vi "pulse_generator_data_v2.vi"(3 "PG Data":refnum<vi>, 4 "Record dP Data":refnum<vi>, 5 "queue in":refnum<queue>, 6 "Stop! Refnum":refnum<vi>, 7 "Recording Progressbar":refnum<vi>, 8 "Seesion Start Time":timestamp, 9 "Pulse Generator Chart Refnums":T3, 10 "Pulse Generator Offsets and Data Saving Controls Refnums":T2, 11 "Pulse Generator Measurement Refnums":T1) -> ()   [LabVIEW 2017]
uses:
  pulse_generator_data_charts_refnums.ctl
  pulse_generator_data_controls_refnums.ctl
  pulse_generator_data_refnums.ctl
  <vilib>/Waveform/WDTOps.llb/WDT Get Waveform Time Array DBL.vi
panel:
  out "size(s)":i32[](graph)
  out "Sampling Rate":refnum<vi>
  out "Recording Duration":refnum<vi>
  out "Camera Voltage Chart":refnum<vi>
  out "Abs Tank Pressure Chart":refnum<vi>
  out "Pitot dP Chart":refnum<vi>
  out "Pulse Generator to Test Section dP Chart":refnum<vi>
  out "W1-7 dP":refnum<vi>
  out "W1-4 dP":refnum<vi>
  out "Mass Flow Rate":refnum<vi>
  out "Liquid Sat Pressure":refnum<vi>
  out "Liquid Temperature":refnum<vi>
  out "Vapor Sat Pressure":refnum<vi>
  out "Vapor Temperature":refnum<vi>
  out "Pitot dP":refnum<vi>
  out "PG to TS dP":refnum<vi>
  out "Pitot Current":refnum<vi>
  out "PG Abs Pressure":refnum<vi>
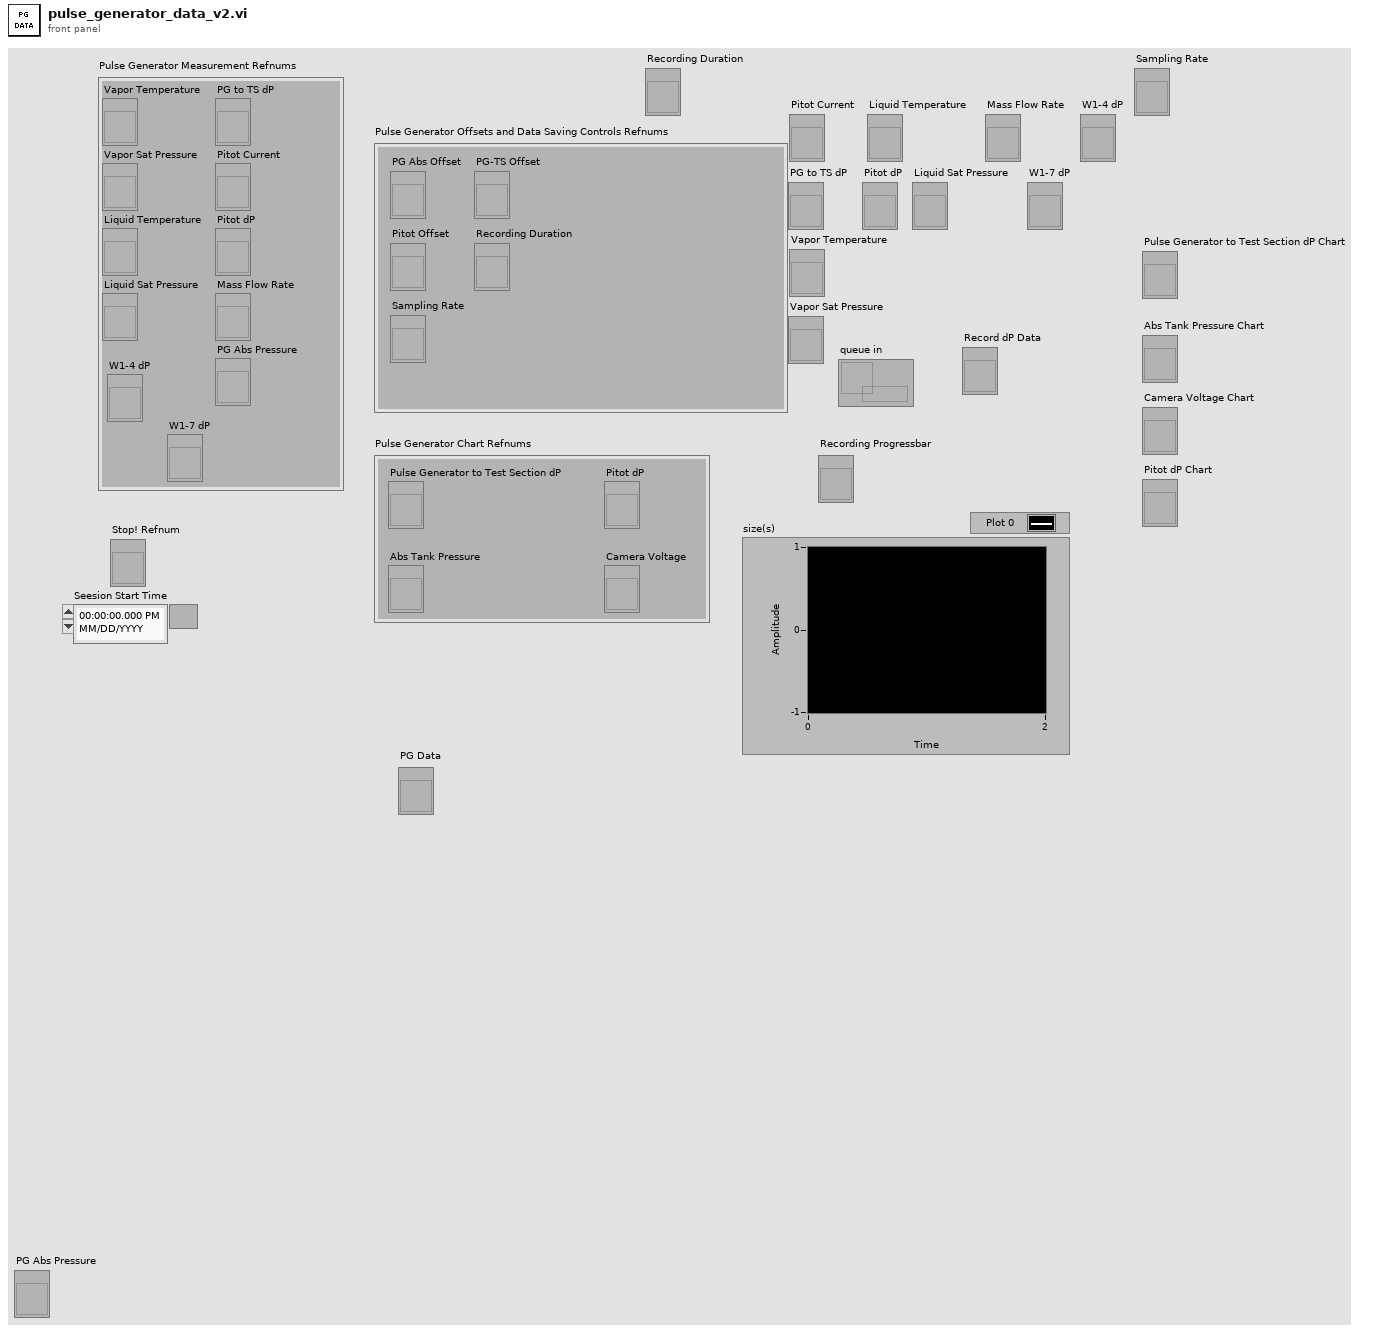
[diagram p1: front panel]
types:
  T1 = typedef "pulse_generator_data_refnums.ctl" = cluster{"Vapor Temperature":refnum<vi>, "Vapor Sat Pressure":refnum<vi>, "Liquid Temperature":refnum<vi>, "Liquid Sat Pressure":refnum<vi>, "PG to TS dP":refnum<vi>, "Pitot Current":refnum<vi>, "Pitot dP":refnum<vi>, "Mass Flow Rate":refnum<vi>, "PG Abs Pressure":refnum<vi>, "W1-4 dP":refnum<vi>, "W1-7 dP":refnum<vi>}
  T2 = typedef "pulse_generator_data_controls_refnums.ctl" = cluster{"PG Abs Offset":refnum<vi>, "Pitot Offset":refnum<vi>, "PG-TS Offset":refnum<vi>, "Recording Duration":refnum<vi>, "Sampling Rate":refnum<vi>}
  T3 = typedef "pulse_generator_data_charts_refnums.ctl" = cluster{"Pulse Generator to Test Section dP":refnum<vi>, "Pitot dP":refnum<vi>, "Abs Tank Pressure":refnum<vi>, "Camera Voltage":refnum<vi>}
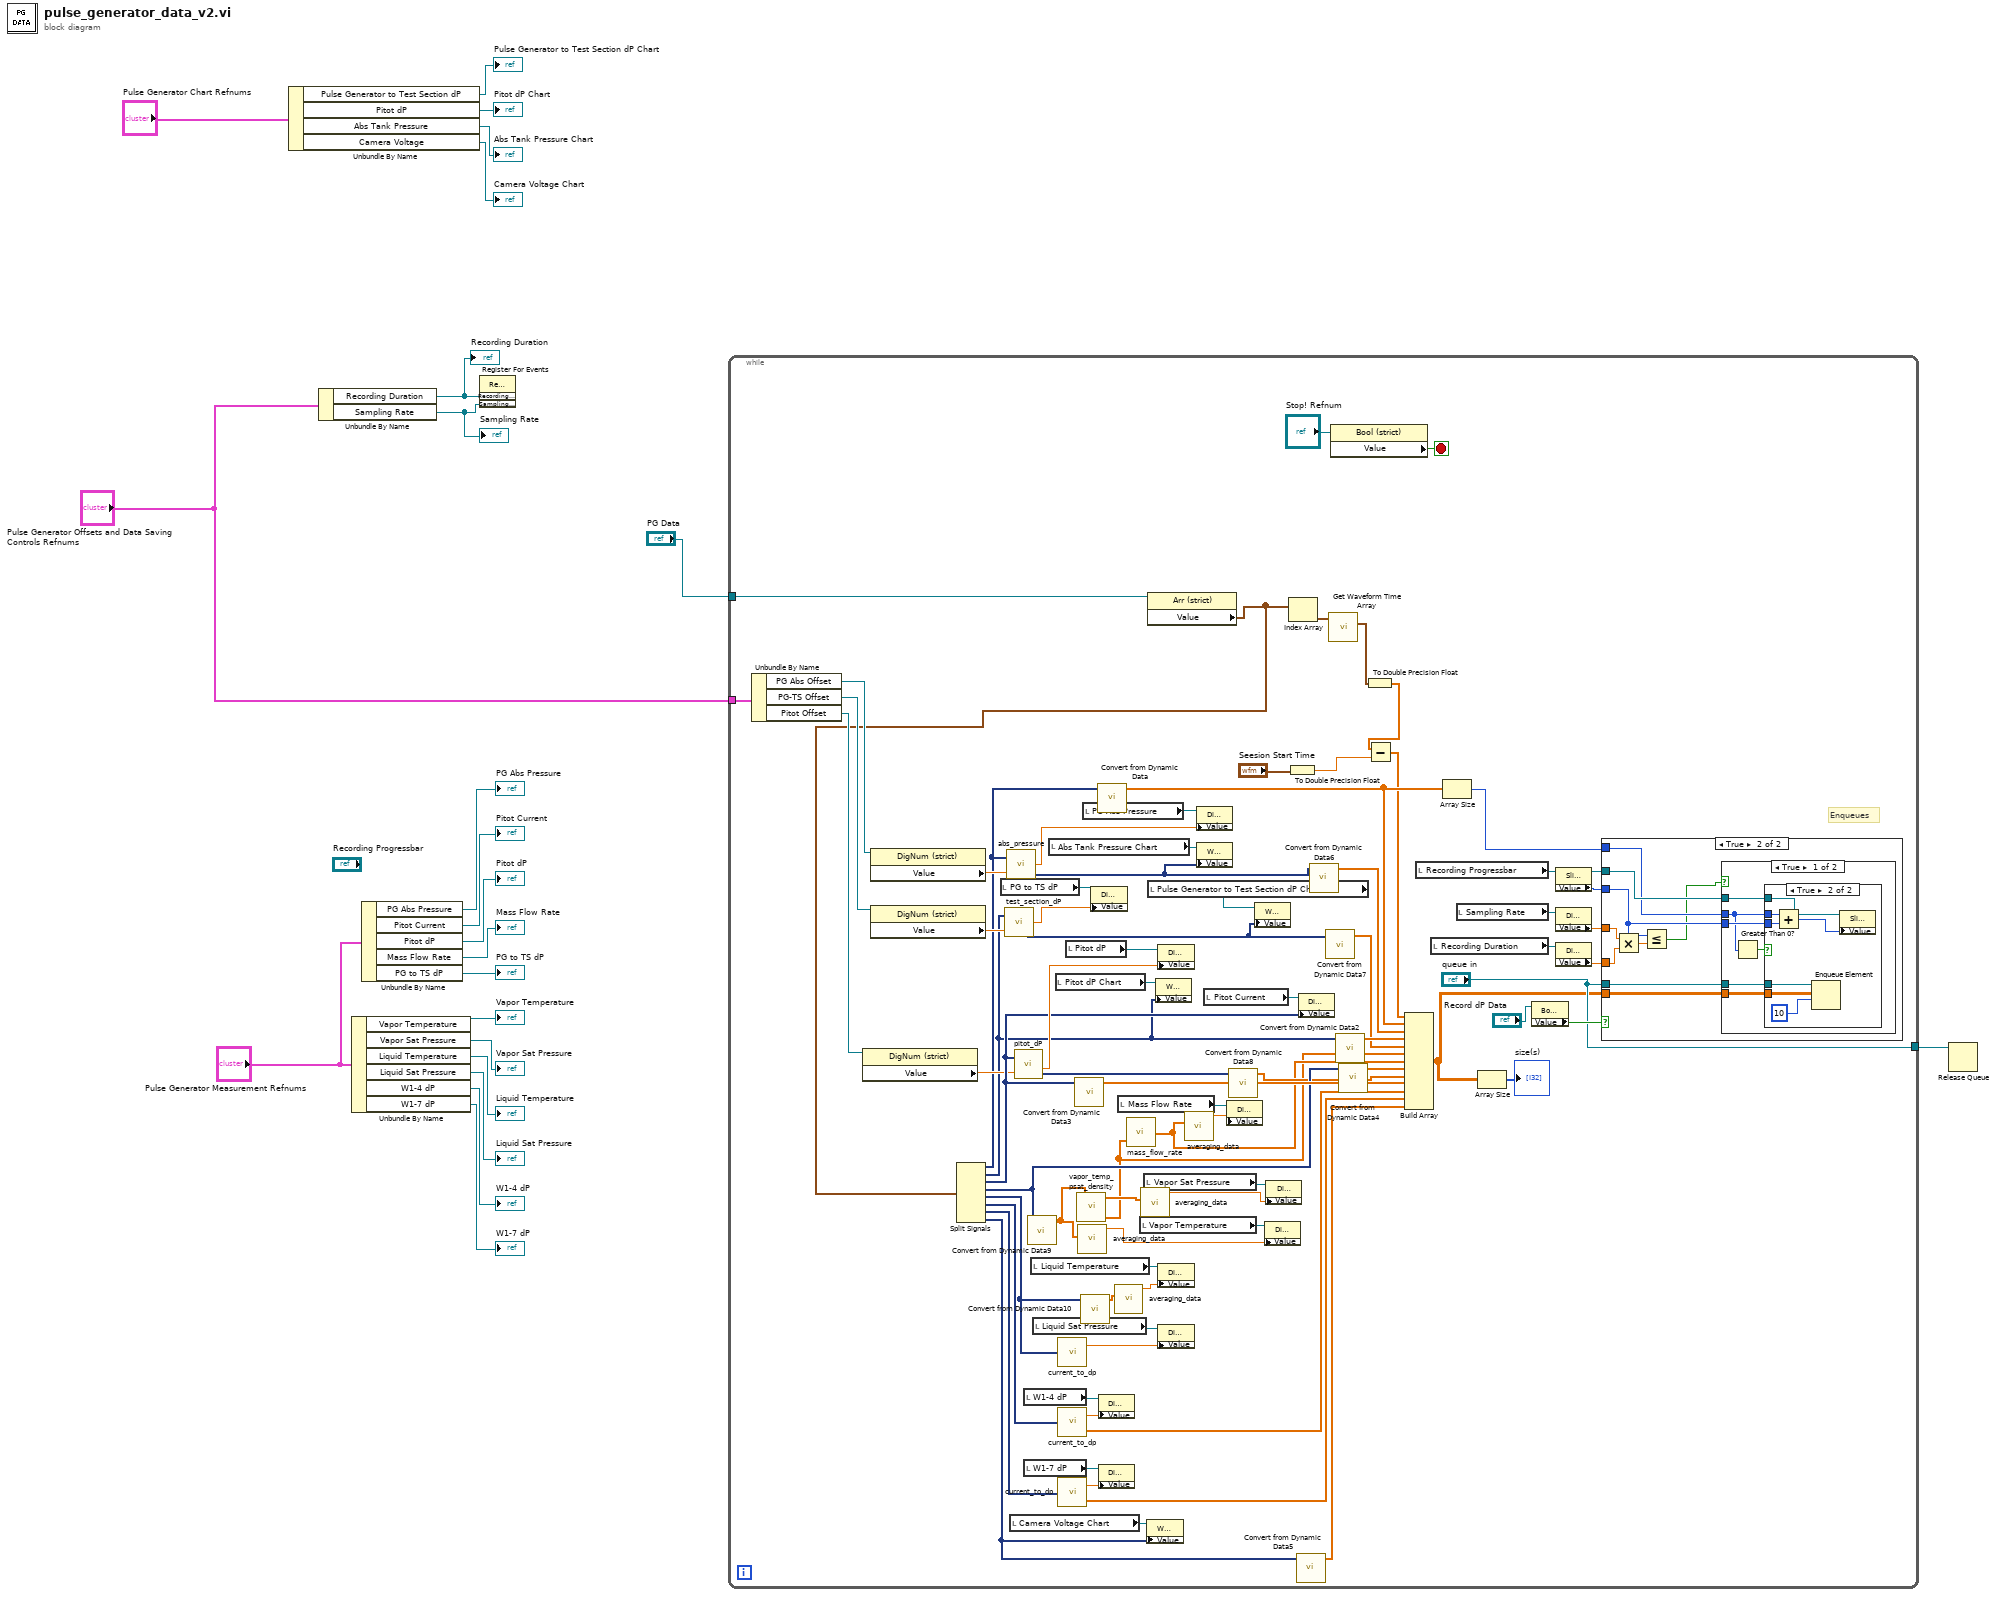
[diagram p0: block diagram]
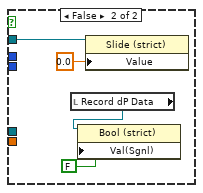
[diagram p4: hidden frame]
diagram:
  n1 = Unbundle By Name("Pulse Generator Chart Refnums") -> ("Pulse Generator to Test Section dP"=→"Pulse Generator to Test Section dP Chart":refnum<vi>, "Pitot dP"=→"Pitot dP Chart":refnum<vi>, "Abs Tank Pressure"=→"Abs Tank Pressure Chart":refnum<vi>, "Camera Voltage"=→"Camera Voltage Chart":refnum<vi>)
  n2 = Unbundle By Name("Pulse Generator Offsets and Data Saving Controls Refnums") -> ("Recording Duration"=w4:refnum<vi>, "Sampling Rate"=w3:refnum<vi>)
  "Recording Duration" <- w4
  "Sampling Rate" <- w3
  n3 = Unbundle By Name("Pulse Generator Measurement Refnums") -> ("Vapor Temperature"=→"Vapor Temperature":refnum<vi>, "Vapor Sat Pressure"=→"Vapor Sat Pressure":refnum<vi>, "Liquid Temperature"=→"Liquid Temperature":refnum<vi>, "Liquid Sat Pressure"=→"Liquid Sat Pressure":refnum<vi>, "W1-4 dP"=→"W1-4 dP":refnum<vi>, "W1-7 dP"=→"W1-7 dP":refnum<vi>)
  n4 = Unbundle By Name("Pulse Generator Measurement Refnums") -> ("PG Abs Pressure"=→"PG Abs Pressure":refnum<vi>, "Pitot Current"=→"Pitot Current":refnum<vi>, "Pitot dP"=→"Pitot dP":refnum<vi>, "Mass Flow Rate"=→"Mass Flow Rate":refnum<vi>, "PG to TS dP"=→"PG to TS dP":refnum<vi>)
  n5 = register-events(w4, w3) -> ()  [unwired: 2 in, 2 out]
  n6 = while {
    tunnel: "Pulse Generator Offsets and Data Saving Controls Refnums" -> [w101]
    tunnel: ["queue in"] -> w6
    tunnel: "PG Data" -> [w34]
    stop <- w102 stop-if-true
    # "Enqueues"
    n7 = Unbundle By Name(w101) -> ("PG Abs Offset"=w100:refnum<vi>, "PG-TS Offset"=w99:refnum<vi>, "Pitot Offset"=w98:refnum<vi>)
    n8 = property class="DigNum (strict)"(reference=w98) -> ("Value"=w52:dbl)  [unwired: 1 in, 2 out]
    n9 = property class="DigNum (strict)"(reference=w100) -> ("Value"=w97:dbl)  [unwired: 1 in, 2 out]
    n10 = property class="DigNum (strict)"(reference=w99) -> ("Value"=w56:dbl)  [unwired: 1 in, 2 out]
    n11 = local read "PG to TS dP"() -> (w96:refnum<vi>)
    n12 = local read "Camera Voltage Chart"() -> (w77:refnum<vi>)
    n13 = local read "W1-4 dP"() -> (w87:refnum<vi>)
    n14 = local read "W1-7 dP"() -> (w84:refnum<vi>)
    n15 = local read "Liquid Temperature"() -> (w90:refnum<vi>)
    n16 = local read "Liquid Sat Pressure"() -> (w92:refnum<vi>)
    n17 = local read "Abs Tank Pressure Chart"() -> (w80:refnum<vi>)
    n18 = local read "Pitot dP Chart"() -> (w79:refnum<vi>)
    n19 = local read "Pitot dP"() -> (w94:refnum<vi>)
    n20 = local read "PG Abs Pressure"() -> (w54:refnum<vi>)
    n21 = local read "Mass Flow Rate"() -> (w93:refnum<vi>)
    n22 = local read "Vapor Temperature"() -> (w89:refnum<vi>)
    n23 = local read "Vapor Sat Pressure"() -> (w82:refnum<vi>)
    n24 = property class="Arr (strict)"(reference=w34) -> ("Value"=w33:waveform(dbl)[])  [unwired: 1 in, 2 out]
    n25 = Split Signals(w33) -> (w41:dynamicdata, w50:dynamicdata, w59:dynamicdata, w57:dynamicdata, w28:dynamicdata, w86:dynamicdata, w85:dynamicdata, w68:dynamicdata)  [unwired: 8 in]
    n26 = call "test_section_dP.vi"("dP Voltage"=w50, "Offset[Pa]"=w56) -> ("Adj dP"=w75:dbl, "Adj dP Array"=w44:dynamicdata)  [unwired: 1 out]
    n27 = call "abs_pressure.vi"("Input Voltage"=w41, "Offset[Pa]"=w97) -> ("Adj Absolute Pressure"=w76:dbl, "Adj Absolute Pressure Array"=w46:dynamicdata)  [unwired: 1 out]
    n28 = call "pitot_dP.vi"("Pitot Current"=w59, "Pitot Offset [Pa]"=w52) -> ("Adj dP [Pa]"=w78:dbl, "Adj dP [Pa] Array"=w42:dynamicdata)  [unwired: 2 out]
    n29 = call "Convert from Dynamic Data9"("Dynamic Data Type"=w57) -> ("Array"=w32:dbl[])  [unwired: 3 in]
    n30 = call "current_to_dp.vi"("Current [A]"=w28) -> ("dP [Pa]"=w91:dbl)  [unwired: 1 out]
    n31 = call "current_to_dp.vi"("Current [A]"=w86) -> ("dP [Pa]"=w88:dbl, "dP Array [Pa]"=w74:dbl[])
    n32 = call "current_to_dp.vi"("Current [A]"=w85) -> ("dP [Pa]"=w83:dbl, "dP Array [Pa]"=w58:dbl[])
    n33 = call "Convert from Dynamic Data3"("Dynamic Data Type"=w59) -> ("Array"=w71:dbl[])  [unwired: 3 in]
    n34 = call "vapor_temp_psat_density.vi"("Vapor Temp [C]"=w32) -> ("Psat Vapor"=w30:dbl[], "Vapor Density"=w23:dbl[])  [unwired: 1 in]
    n35 = call "averaging_data.vi"("Input"=w32) -> ("Average"=w31:dbl)  [unwired: 6 in, 3 out]
    n36 = call "Convert from Dynamic Data10"("Dynamic Data Type"=w28) -> ("Array"=w27:dbl[])  [unwired: 3 in]
    n37 = property class="DigNum (strict)"(reference=w96, "Value"=w75) -> ()  [unwired: 1 in, 2 out]
    n38 = call "Convert from Dynamic Data"("Dynamic Data Type"=w41) -> ("Array"=w67:dbl[])  [unwired: 3 in]
    n39 = property class="DigNum (strict)"(reference=w87, "Value"=w88) -> ()  [unwired: 1 in, 2 out]
    n40 = property class="DigNum (strict)"(reference=w84, "Value"=w83) -> ()  [unwired: 1 in, 2 out]
    n41 = call "averaging_data.vi"("Input"=w27) -> ("Average"=w26:dbl)  [unwired: 6 in, 3 out]
    n42 = call "mass_flow_rate.vi"("Density"=w23) -> ("Mass Flow Rate [g/s] Array"=w25:dbl[])  [unwired: 1 in]
    n43 = call "averaging_data.vi"("Input"=w30) -> ("Average"=w29:dbl)  [unwired: 6 in, 3 out]
    n44 = property class="WFChart (strict)"(reference=w77, "Value"=w68) -> ()  [unwired: 1 in, 2 out]
    n45 = local read "Pulse Generator to Test Section dP Chart"() -> (w81:refnum<vi>)
    n46 = property class="WFChart (strict)"(reference=w79, "Value"=w50) -> ()  [unwired: 1 in, 2 out]
    n47 = property class="DigNum (strict)"(reference=w94, "Value"=w78) -> ()  [unwired: 1 in, 2 out]
    n48 = property class="DigNum (strict)"(reference=w90, "Value"=w26) -> ()  [unwired: 1 in, 2 out]
    n49 = property class="DigNum (strict)"(reference=w92, "Value"=w91) -> ()  [unwired: 1 in, 2 out]
    n50 = call "averaging_data.vi"("Input"=w25) -> ("Average"=w24:dbl)  [unwired: 6 in, 3 out]
    n51 = property class="DigNum (strict)"(reference=w54, "Value"=w76) -> ()  [unwired: 1 in, 2 out]
    n52 = property class="WFChart (strict)"(reference=w80, "Value"=w46) -> ()  [unwired: 1 in, 2 out]
    n53 = local read "Pitot Current"() -> (w95:refnum<vi>)
    n54 = property class="DigNum (strict)"(reference=w93, "Value"=w24) -> ()  [unwired: 1 in, 2 out]
    n55 = call "Convert from Dynamic Data8"("Dynamic Data Type"=w42) -> ("Array"=w43:dbl[])  [unwired: 3 in]
    n56 = property class="WFChart (strict)"(reference=w81, "Value"=w44) -> ()  [unwired: 1 in, 2 out]
    n57 = property class="DigNum (strict)"(reference=w89, "Value"=w31) -> ()  [unwired: 1 in, 2 out]
    n58 = property class="DigNum (strict)"(reference=w82, "Value"=w29) -> ()  [unwired: 1 in, 2 out]
    n59 = To Double Precision Float(number="Seesion Start Time") -> (double precision float=w36:dbl)
    n60 = Index Array(array=w33) -> (element=w40:waveform(dbl))  [unwired: 1 in]
    n61 = call "Convert from Dynamic Data5"("Dynamic Data Type"=w68) -> ("Array"=w69:dbl[])  [unwired: 3 in]
    n62 = property class="DigNum (strict)"(reference=w95, "Value"=w59) -> ()  [unwired: 1 in, 2 out]
    n63 = call "Convert from Dynamic Data6"("Dynamic Data Type"=w46) -> ("Array"=w47:dbl[])  [unwired: 3 in]
    n64 = call "Convert from Dynamic Data7"("Dynamic Data Type"=w44) -> ("Array"=w45:dbl[])  [unwired: 3 in]
    n65 = call-poly <vilib>:"Get Waveform Time Array.vi"("waveform in"=w40) -> ("X array"=w39:timestamp[])  [unwired: 9 in, 1 out]
    n66 = property class="Bool (strict)"(reference="Stop! Refnum") -> ("Value"=w102:bool)  [unwired: 1 in, 2 out]
    n67 = call "Convert from Dynamic Data2"("Dynamic Data Type"=w50) -> ("Array"=w72:dbl[])  [unwired: 3 in]
    n68 = call "Convert from Dynamic Data4"("Dynamic Data Type"=w57) -> ("Array"=w70:dbl[])  [unwired: 3 in]
    n69 = To Double Precision Float(number=w39) -> (double precision float=w38:dbl[])
    n70 = Subtract(x=w38, y=w36) -> (x-y=w35:dbl[])
    n71 = Build Array(w35, w67, w47, w72, w45, w23, w25, w70, w43, w71, w74, w58, w69) -> (w49:dbl[][])
    n72 = local read "Recording Progressbar"() -> (w61:refnum<vi>)
    n73 = local read "Recording Duration"() -> (w65:refnum<vi>)
    n74 = Array Size(array=w67) -> (size(s)=w53:i32)
    n75 = local read "Sampling Rate"() -> (w66:refnum<vi>)
    n76 = Array Size(array=w49) -> (size(s)=→"size(s)":i32[])
    n77 = property class="Bool (strict)"(reference="Record dP Data") -> ("Value"=w55:bool)  [unwired: 1 in, 2 out]
    n78 = property class="Slide (strict)"(reference=w61) -> (reference out=w60:refnum<vi>, "Value"=w62:u32)  [unwired: 1 in, 1 out]
    n79 = property class="DigNum (strict)"(reference=w66) -> ("Value"=w64:dbl)  [unwired: 1 in, 2 out]
    n80 = property class="DigNum (strict)"(reference=w65) -> ("Value"=w63:dbl)  [unwired: 1 in, 2 out]
    n81 = case shown="True" w55 {
      tunnel: "queue in" -> [_ w112]
      tunnel: w53 -> [_ w105]
      tunnel: w64 -> [_ w111]
      tunnel: w63 -> [_ w110]
      tunnel: w62 -> [_ w108]
      tunnel: w60 -> [_ w107]
      tunnel: w49 -> [_ w106]
      frame False {
      }
      frame True {
        n82 = Multiply(x=w111, y=w110) -> (x*y=w109:dbl)
        n83 = Less Or Equal?(x=w108, y=w109) -> (x <= y?=w104:bool)
        n84 = case shown="True" w104 {
          tunnel: w112 -> [w118 _]
          tunnel: w107 -> [w117 w129]
          tunnel: w108 -> [w116 _]
          tunnel: w105 -> [w113 _]
          tunnel: w106 -> [w115 _]
          frame True {
            n85 = Greater Than 0?(x=w113) -> (x > 0?=w114:bool)
            n86 = case shown="True" w114 {
              tunnel: w118 -> [_ w124]
              tunnel: w117 -> [_ w123]
              tunnel: w116 -> [_ w121]
              tunnel: w113 -> [_ w120]
              tunnel: w115 -> [_ w119]
              frame False {
              }
              frame True {
                n87 = Add(x=w120, y=w121) -> (x+y=w122:u32)
                n88 = Enqueue Element(queue=w124, element=w119, timeout in ms (-1)=10) -> ()  [unwired: 1 in, 3 out]
                n89 = property class="Slide (strict)"(reference=w123, "Value"=w122) -> ()  [unwired: 1 in, 2 out]
              }
            }
          }
          frame False {
            n90 = local read "Record dP Data"() -> (w126:refnum<vi>)
            n91 = property class="Bool (strict)"(reference=w126, "Val(Sgnl)"=FALSE ("Value (Signaling)")) -> ()  [unwired: 1 in, 2 out]
            n92 = property class="Slide (strict)"(reference=w129, "Value"=0.0) -> ()  [unwired: 1 in, 2 out]
          }
        }
      }
    }
  }
  n93 = Release Queue(queue=w6) -> ()  [unwired: 2 in, 3 out]
